vi "Take Image Case Struct.vi"(8 "error in (no error)":errorcluster, 9 "OK Button":bool, 10 "Image In":T1, 11 "Session In":T2) -> (0 "error out":errorcluster, 1 "State":string, 2 "Image Out":T1, 3 "Session Out":T2)   [LabVIEW 2024]
uses:
  <vilib>/userDefined/High Color/IMAQdx.ctl
  <vilib>/vision/Image Controls.llb/IMAQ Image.ctl
  <vilib>/vision/driver/IMAQdx.llb/IMAQdx Buffer Number Mode.ctl
  <vilib>/vision/driver/NI_Vision_Acquisition_Software.lvlib
panel:
  # "Input Elements"
  # "Control Elements"
  # "Output Elements"
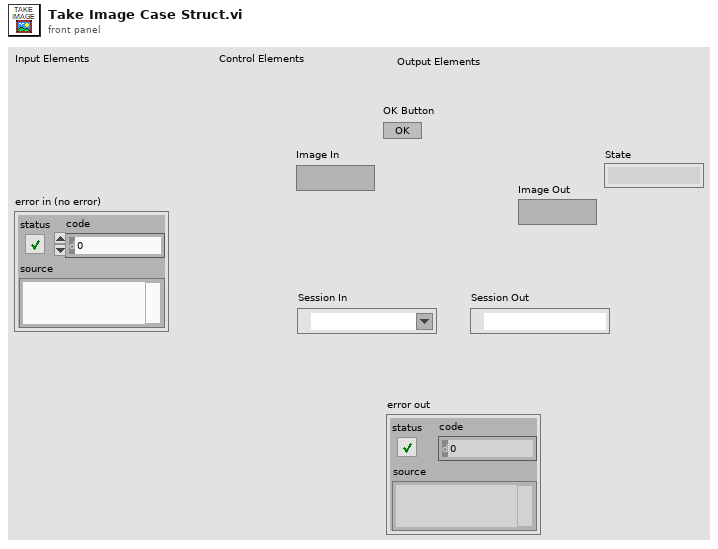
[diagram p1: front panel]
types:
  T1 = typedef "IMAQ Image.ctl" = refnum<image>
  T2 = typedef "IMAQdx.ctl" = refnum<k21>
  T3 = typedef "NI_Vision_Acquisition_Software.lvlib/IMAQdx Buffer Number Mode.ctl" = enum32{"Next", "Last", "Buffer Number", "Every", "Last New"}
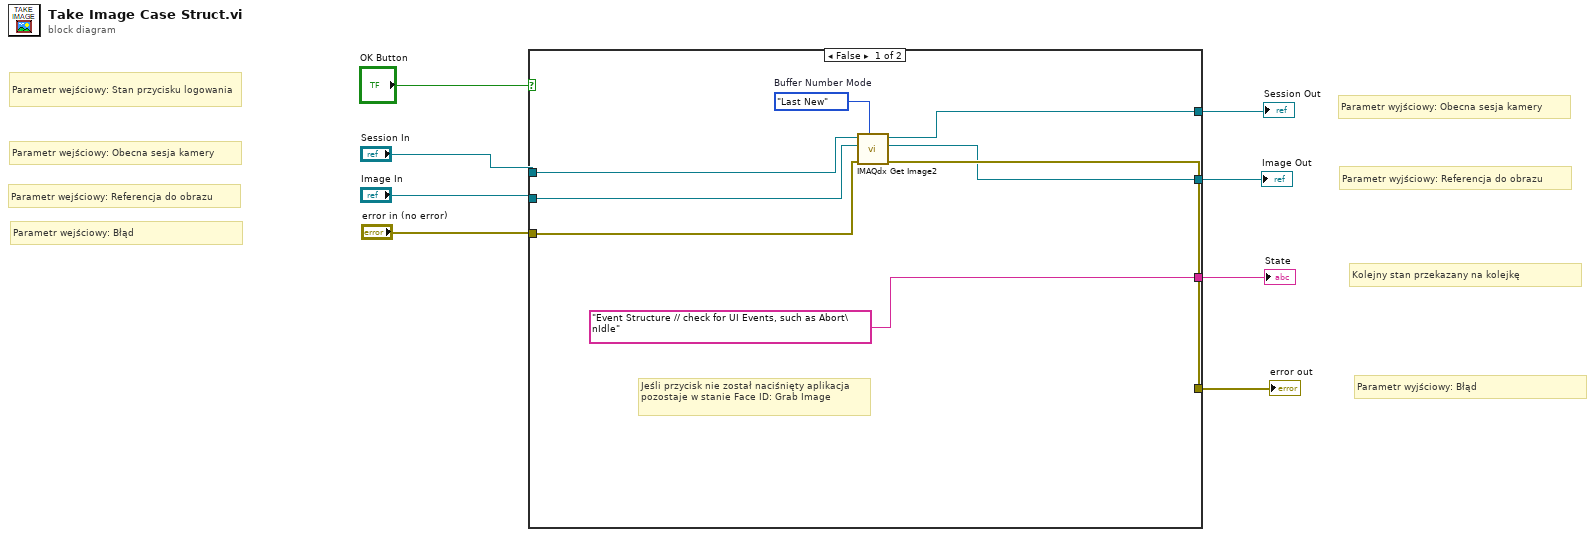
[diagram p0: block diagram]
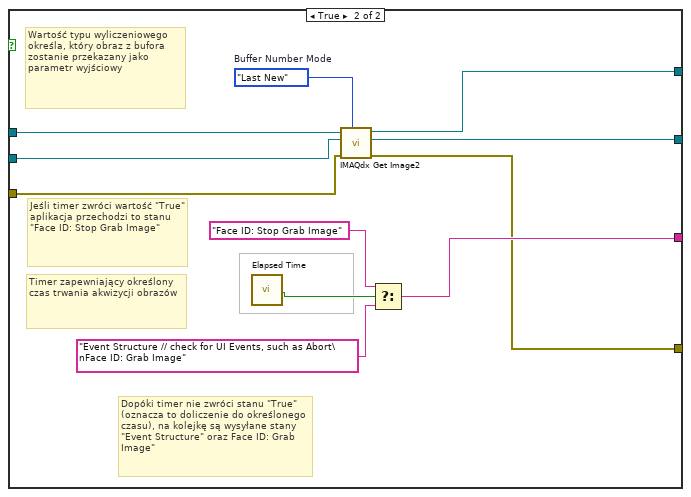
[diagram p2: hidden frame]
diagram:
  # "Parametr wejściowy: Błąd"
  # "Parametr wejściowy: Referencja do obrazu"
  # "Parametr wejściowy: Obecna sesja kamery"
  # "Parametr wejściowy: Stan przycisku logowania"
  # "Parametr wyjściowy: Błąd"
  # "Kolejny stan przekazany na kolejkę"
  # "Parametr wyjściowy: Referencja do obrazu"
  # "Parametr wyjściowy: Obecna sesja kamery"
  n1 = case shown="False" "OK Button" {
    tunnel: [w16 w20] -> w6
    tunnel: ["Event Structure // check for UI Events, such as Abort\nIdle" ("f") w22] -> w1
    tunnel: "Session In" -> [w13 w24]
    tunnel: "Image In" -> [w12 w23]
    tunnel: "error in (no error)" -> [w11 w21]
    tunnel: [w14 w18] -> w3
    tunnel: [w10 w17] -> w2
    frame False {
      w15 = IMAQdx_Buffer_Number_Mode."Last New"  # Buffer Number Mode
      # "Jeśli przycisk nie został naciśnięty aplikacja pozostaje w stanie Face ID: Grab Image"
      n2 = call <vilib>:"IMAQdx Get Image2.vi"("Buffer Number Mode (Next)"=w15, "error in"=w11, "Image In"=w12, "Session In"=w13) -> ("error out"=w16:errorcluster, "Image Out"=w14:T1, "Session Out"=w10:T2)  [unwired: 4 in, 1 out]
    }
    frame True {
      w19 = IMAQdx_Buffer_Number_Mode."Last New"  # Buffer Number Mode
      # "Wartość typu wyliczeniowego określa, który obraz z bufora zostanie przekazany jako parametr wyjściowy"
      # "Jeśli timer zwróci wartość \"True\" aplikacja przechodzi to stanu \"Face ID: Stop Grab Image\""
      # "Dopóki timer nie zwróci stanu \"True\" (oznacza to doliczenie do określonego czasu), na kolejkę są wysyłane stany \"Event Structure\" oraz Face ID: Grab Image\""
      # "Timer zapewniający określony czas trwania akwizycji obrazów"
      n3 = call "Elapsed Time"() -> ("Time has Elapsed"=w27:bool)  [unwired: 12 in, 7 out]
      n4 = call <vilib>:"IMAQdx Get Image2.vi"("Buffer Number Mode (Next)"=w19, "error in"=w21, "Image In"=w23, "Session In"=w24) -> ("error out"=w20:errorcluster, "Image Out"=w18:T1, "Session Out"=w17:T2)  [unwired: 4 in, 1 out]
      n5 = Select(t="Face ID: Stop Grab Image", s=w27, f="Event Structure // check for UI Events, such as Abort\nFace ID: Grab Image") -> (s? t:f=w22:string)
    }
  }
  "error out" <- w6
  "Session Out" <- w2
  "Image Out" <- w3
  "State" <- w1
